vi "Hauptprogramm.vi"() -> ()   [LabVIEW 2021]
uses:
  Global Variabeln.vi
panel:
  in  "min. Zeit\n zwischen Daten [s]":dbl
  out "XY Graph":cluster{timestamp[], dbl[]}[](graph)
  out "aktuell Daten Schreiben":bool
  out "Aktuelle\nLuftfeuchtigkeit":dbl(knob) scale=0.0..100.0
  out "Aktuelle \nTemperatur":dbl(slide) scale=-10.0..40.0
  out "Aktuell Diagramm":bool
  out "Aktuell Laufschrift \nZeit":bool
  out "Aktuell Laufschrift\nHum+Temp":bool
  in  "Diagramm":bool=TRUE
  in  "Laufschrift\nZeit":bool=TRUE
  in  "Laufschrift\nTemperatur\nu.\nHumluftfeuchtigkeit":bool=TRUE
  in  "Daten \nschreiben":bool=TRUE
  in  "Helligkeit der \nLED's [%]":dbl(knob) min=0.0 max=100.0 step=1.0 scale=0.0..100.0
  in  "stop":bool
  in  "VISA resource name":refnum<visa-resource-name>
  out "Color Box 2":u32(colorbox)=11316396
  # "Aktueller\nState"
  # "State \nÜberspringen"
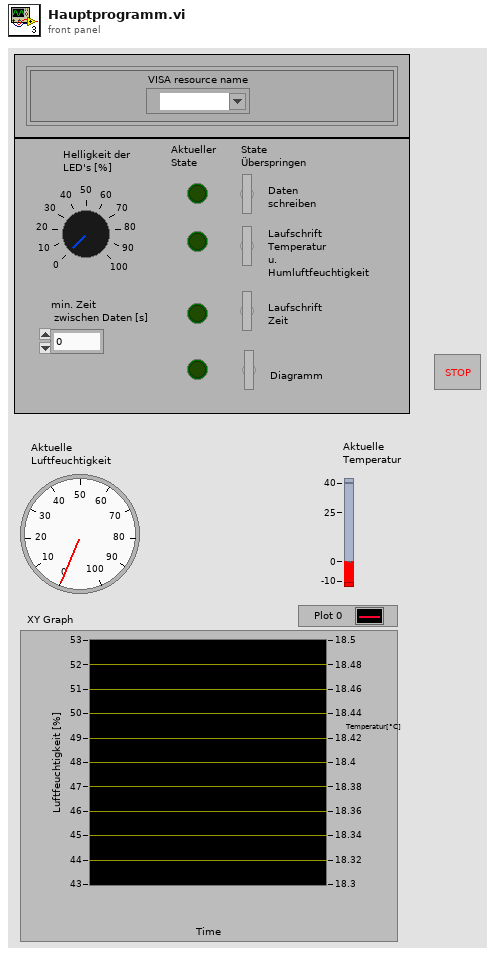
[diagram p1: front panel]
types:
  T1 = enum16{"Init", "Daten Schreiben", "Laufschrift Temp+Hum", "Laufschrift Zeit+Date", "Diagramm Plotten"}
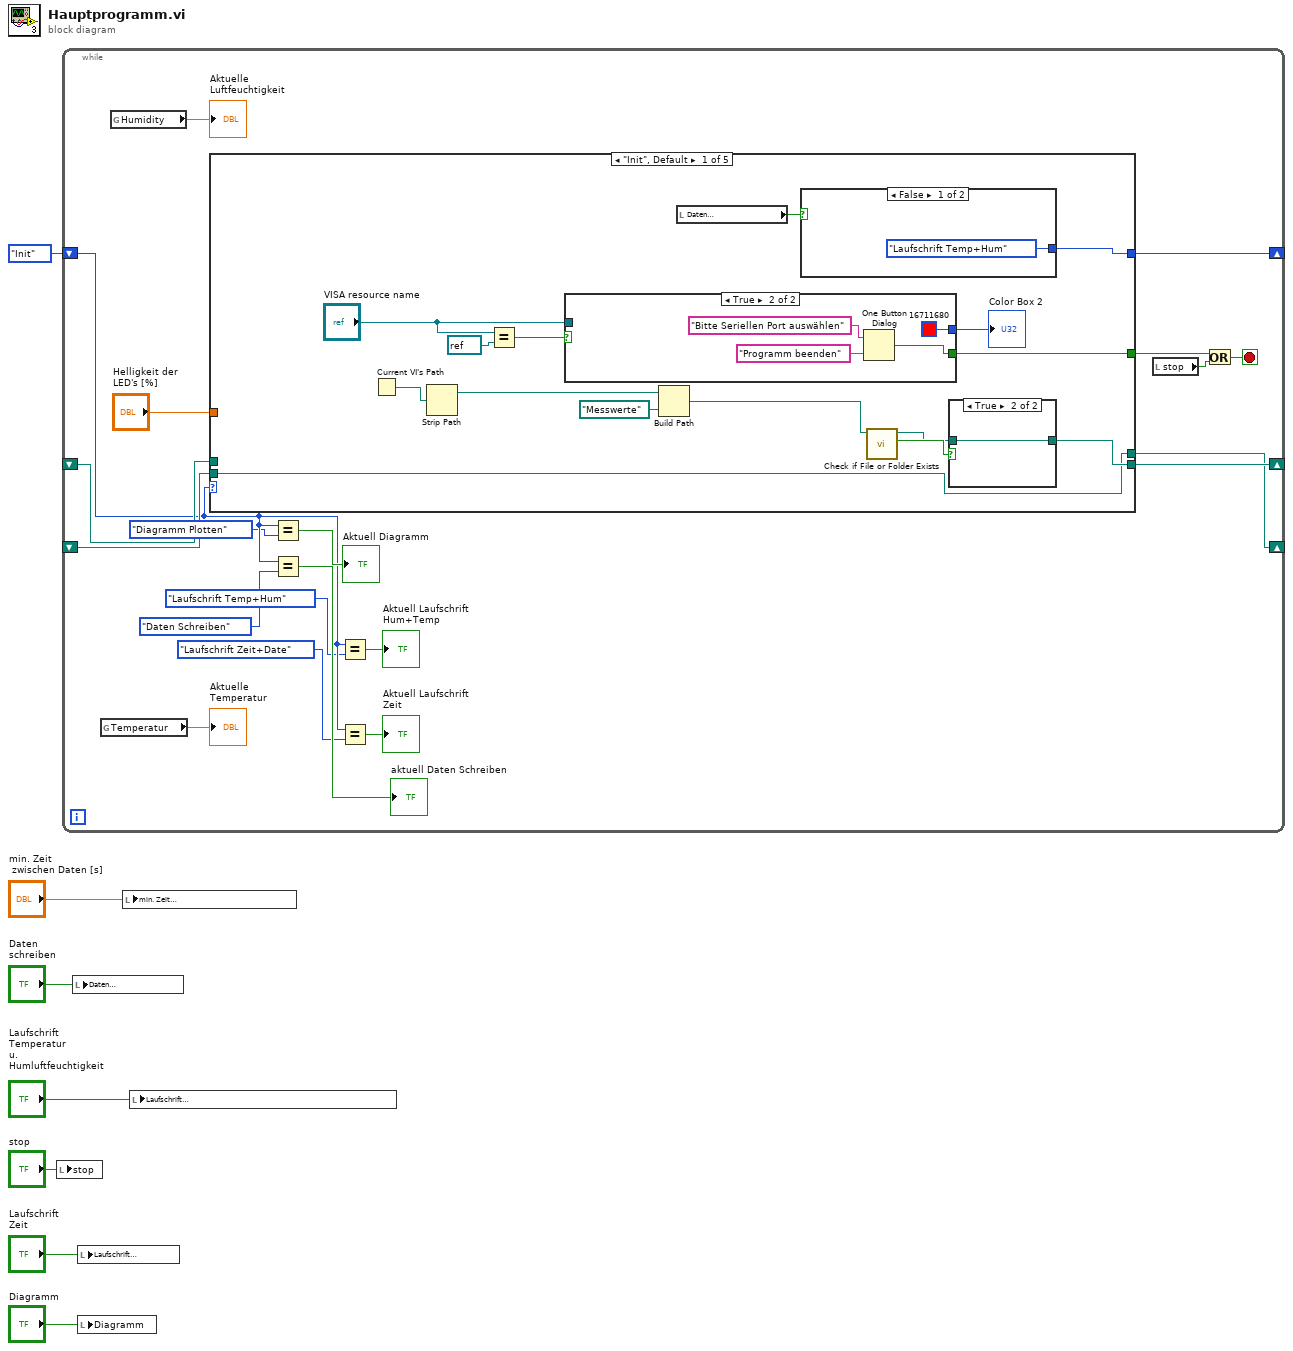
[diagram p0: block diagram]
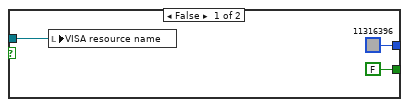
[diagram p2: hidden frame]
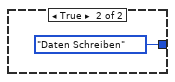
[diagram p3: hidden frame]
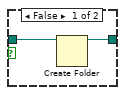
[diagram p4: hidden frame]
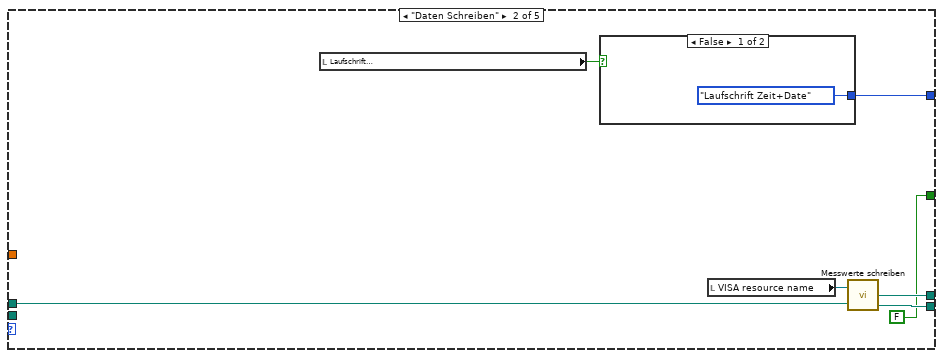
[diagram p5: hidden frame]
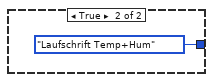
[diagram p6: hidden frame]
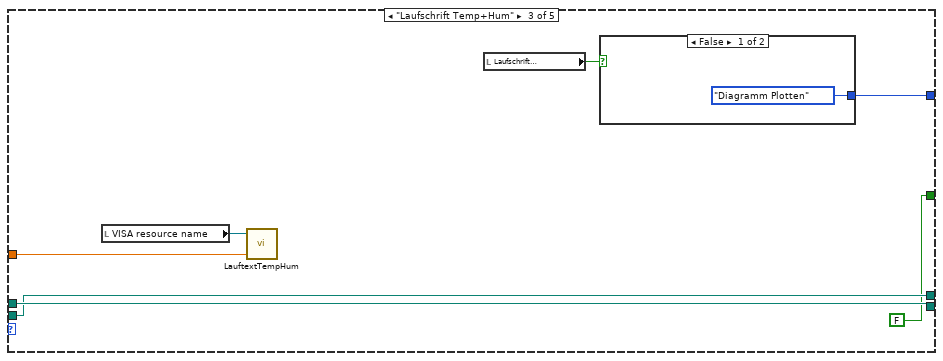
[diagram p7: hidden frame]
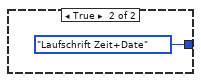
[diagram p8: hidden frame]
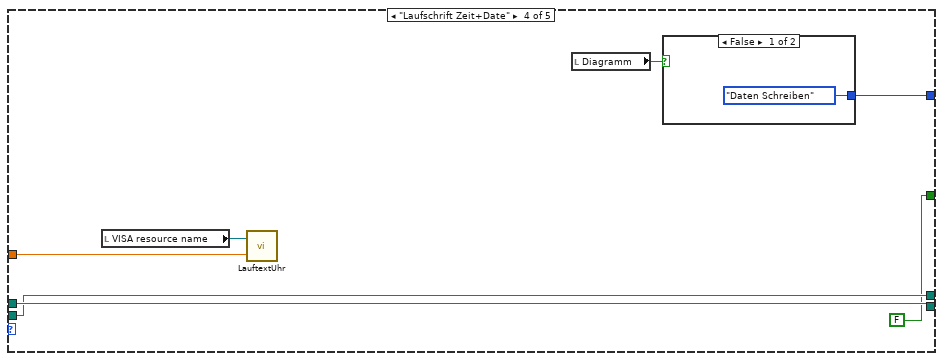
[diagram p9: hidden frame]
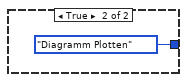
[diagram p10: hidden frame]
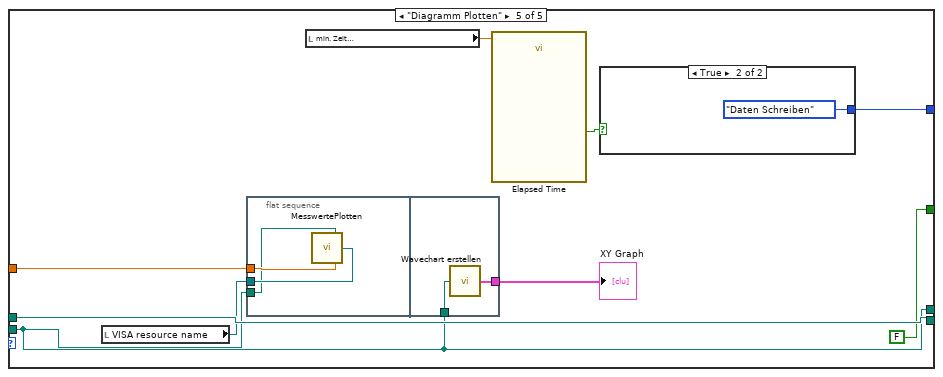
[diagram p11: hidden frame]
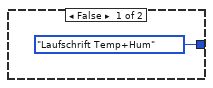
[diagram p12: hidden frame]
diagram:
  n1 = local write "stop"("stop") -> ()
  n2 = while {
    shift-right: [w26] -> _
    shift-left: _ -> [w27]
    shift-right: [w20] -> _
    shift-left: T1."Init" ("Enum") -> [w15]
    shift-right: [w25] -> _
    shift-left: _ -> [w24]
    stop <- w10 stop-if-true
    n3 = global read "Global Variabeln.vi" "Temperatur"() -> (→"Aktuelle \nTemperatur":dbl)
    n4 = global read "Global Variabeln.vi" "Humidity"() -> (→"Aktuelle\nLuftfeuchtigkeit":dbl)
    n5 = case shown="\"Init\", Default" w15 {
      tunnel: [w41 w61 w69 w77 w90] -> w26
      tunnel: [w38 w57 w66 w78 w84] -> w20
      tunnel: "Helligkeit der \nLED's [%]" -> [_ _ w70 w79 w89]
      tunnel: w27 -> [_ w60 w69 w77 w90]
      tunnel: [w39 w59 w68 w76 w87] -> w25
      tunnel: w24 -> [w39 _ w68 w76 w87]
      tunnel: [w32 FALSE ("true") FALSE ("true") FALSE ("true") FALSE ("true")] -> w8
      frame "Init", Default {
        n6 = Current VI's Path() -> (path=w31:path)
        n7 = Strip Path(path=w31) -> (stripped path=w30:path)  [unwired: 1 out]
        n8 = Equal?(x="VISA resource name", y=refnum<visa-resource-name> refnum) -> (x = y?=w36:bool)
        n9 = case shown="True" w36 {
          tunnel: "VISA resource name" -> [w45 _]
          tunnel: [FALSE w47] -> w32
          tunnel: [u32 11316396 ("Color Box 2") u32 16711680 ("Color Box 2")] -> w33
          frame False {
            n10 = local write "VISA resource name"(w45) -> ()
          }
          frame True {
            n11 = One Button Dialog(message="Bitte Seriellen Port auswählen", button name ("OK")="Programm beenden" ("F button name (\"Cancel\")")) -> (true=w47:bool)
          }
        }
        "Color Box 2" <- w33
        n12 = Build Path(base path=w30, name or relative path=path "Messwerte") -> (appended path=w28:path)
        n13 = local read "Daten \nschreiben"() -> (w37:bool)
        n14 = case shown="False" w37 {
          tunnel: [T1."Laufschrift Temp+Hum" ("Enum") T1."Daten Schreiben" ("Enum")] -> w38
          frame False {
          }
          frame True {
          }
        }
        n15 = call <vilib>:"Check if File or Folder Exists.vi"("path"=w28) -> ("file or folder exists?"=w42:bool, "dup path"=w40:path)  [unwired: 8 in, 1 out]
        n16 = case shown="True" w42 {
          tunnel: [w52 w54] -> w41
          tunnel: w40 -> [w53 w54]
          frame False {
            n17 = Create Folder(path (use dialog)=w53) -> (created path=w52:path)  [unwired: 2 in, 2 out]
          }
          frame True {
          }
        }
      }
      frame "Daten Schreiben" {
        n18 = local read "Laufschrift\nTemperatur\nu.\nHumluftfeuchtigkeit"() -> (w58:bool)
        n19 = case shown="False" w58 {
          tunnel: [T1."Laufschrift Zeit+Date" ("Enum") T1."Laufschrift Temp+Hum" ("Enum")] -> w57
          frame False {
          }
          frame True {
          }
        }
        n20 = local read "VISA resource name"() -> (w56:refnum<visa-resource-name>)
        n21 = call "Messwerte schreiben.vi"("VISA resource name"=w56, "path"=w60) -> ("File Refnumber"=w59:path, "path 2"=w61:path)  [unwired: 1 out]
      }
      frame "Laufschrift Temp+Hum" {
        n22 = local read "VISA resource name"() -> (w65:refnum<visa-resource-name>)
        n23 = call "LauftextTempHum.vi"("Intensity 0-100"=w70, "VISA resource name"=w65) -> ()  [unwired: 1 in, 1 out]
        n24 = local read "Laufschrift\nZeit"() -> (w67:bool)
        n25 = case shown="False" w67 {
          tunnel: [T1."Diagramm Plotten" ("Enum") T1."Laufschrift Zeit+Date" ("Enum")] -> w66
          frame False {
          }
          frame True {
          }
        }
      }
      frame "Laufschrift Zeit+Date" {
        n26 = local read "VISA resource name"() -> (w74:refnum<visa-resource-name>)
        n27 = call "LauftextUhr.vi"("Intensity 0-100"=w79, "VISA resource name"=w74) -> ()  [unwired: 1 out]
        n28 = local read "Diagramm"() -> (w75:bool)
        n29 = case shown="False" w75 {
          tunnel: [T1."Daten Schreiben" ("Enum") T1."Diagramm Plotten" ("Enum")] -> w78
          frame False {
          }
          frame True {
          }
        }
      }
      frame "Diagramm Plotten" {
        n30 = local read "VISA resource name"() -> (w88:refnum<visa-resource-name>)
        n31 = flat-sequence {
          tunnel: w89 -> [w95]
          tunnel: w88 -> [w94]
          tunnel: w87 -> [w93]
          tunnel: w87 -> [w97]
          tunnel: [w96] -> w86
          frame #0 {
            n32 = call "MesswertePlotten.vi"("Intensity 0-100"=w95, "VISA resource name"=w94, "file path (use dialog)"=w93) -> ()  [unwired: 4 in]
          }
          frame #1 {
            n33 = call "Wavechart erstellen.vi"("file path (dialog if empty)"=w97) -> ("XY Graph"=w96:cluster{timestamp[], dbl[]}[])
          }
        }
        n34 = local read "min. Zeit\n zwischen Daten [s]"() -> (w85:dbl)
        n35 = call "Elapsed Time"("Time Target (s)"=w85) -> ("Time has Elapsed"=w82:bool)  [unwired: 11 in, 7 out]
        n36 = case shown="True" w82 {
          tunnel: [T1."Laufschrift Temp+Hum" ("Enum") T1."Daten Schreiben" ("Enum")] -> w84
          frame False {
          }
          frame True {
          }
        }
        "XY Graph" <- w86
      }
    }
    n37 = Equal?(x=w15, y=T1."Diagramm Plotten" ("Enum")) -> (x = y?=→"Aktuell Diagramm":bool)
    n38 = Equal?(x=w15, y=T1."Daten Schreiben" ("Enum")) -> (x = y?=→"aktuell Daten Schreiben":bool)
    n39 = Equal?(x=w15, y=T1."Laufschrift Temp+Hum" ("Enum")) -> (x = y?=→"Aktuell Laufschrift\nHum+Temp":bool)
    n40 = Equal?(x=w15, y=T1."Laufschrift Zeit+Date" ("Enum")) -> (x = y?=→"Aktuell Laufschrift \nZeit":bool)
    n41 = local read "stop"() -> (w9:bool)
    n42 = Or(x=w8, y=w9) -> (x .or. y?=w10:bool)
  }
  n43 = local write "Daten \nschreiben"("Daten \nschreiben") -> ()
  n44 = local write "Laufschrift\nZeit"("Laufschrift\nZeit") -> ()
  n45 = local write "Diagramm"("Diagramm") -> ()
  n46 = local write "min. Zeit\n zwischen Daten [s]"("min. Zeit\n zwischen Daten [s]") -> ()
  n47 = local write "Laufschrift\nTemperatur\nu.\nHumluftfeuchtigkeit"("Laufschrift\nTemperatur\nu.\nHumluftfeuchtigkeit") -> ()
